vi "addBreak.vi"(8 "error in (no error)":errorcluster, 11 "xwpfRun.PageBreak in":refnum<class "xwpfRun.PageBreak.lvclass">) -> (0 "error out":errorcluster, 3 "xwpfRun.PageBreak out":refnum<class "xwpfRun.PageBreak.lvclass">)   [LabVIEW 2017, in "Word_Specific.lvlib" / "xwpfRun.PageBreak.lvclass"]
uses:
  xwpfRun.PageBreak.lvclass
  C:/Users/Neo/Desktop/Dev_Tools_BR/LabVIEW_NPOI/src/LabVIEW NPOI/xwpfRun/xwpfRun.lvclass
  xwpfRun/xwpfRun.lvclass/xwpfRun.ctl
  C:/Users/Neo/Desktop/Dev_Tools_BR/LabVIEW_NPOI/src/lib/NPOI 2.1.1/NPOI.OOXML.dll
  lib/NPOI 2.1.1/NPOI.OOXML.dll
  xwpfRun/Get Run Ref.vi
  xwpfRun.Normal/xwpfRun.Normal.lvclass
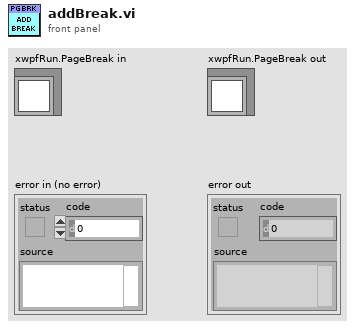
[diagram p1: front panel]
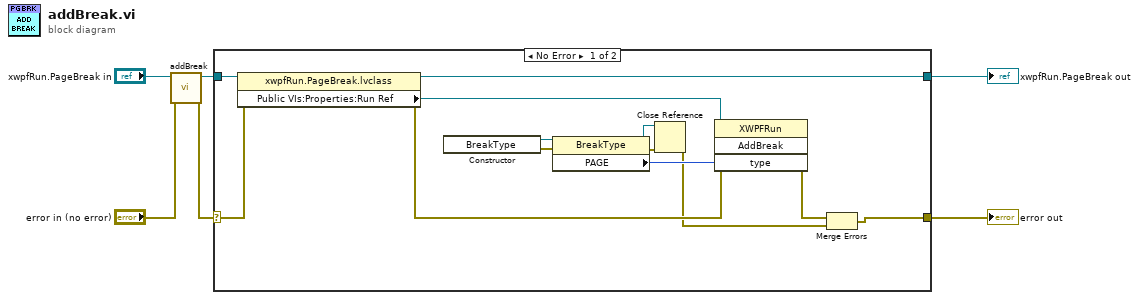
[diagram p0: block diagram]
diagram:
  n1 = call-parent "addBreak.vi"("error in (no error)"="error in (no error)", "xwpfRun in"="xwpfRun.PageBreak in") -> ("error out"=w4:errorcluster, "xwpfRun out"=w2:refnum<class "xwpfRun.PageBreak.lvclass">)  [unwired: 8 in]
  n2 = case shown="No Error" w4 {
    selector: w4 -> [w17 w21]
    tunnel: [w8 w21] -> w3
    tunnel: w2 -> [w19 w20]
    tunnel: [w18 w20] -> w1
    frame No Error {
      n3 = property class="xwpfRun.PageBreak.lvclass"(reference=w19, error in=w17) -> (reference out=w18:refnum<class "xwpfRun.PageBreak.lvclass">, error out=w15:errorcluster, "Public VIs:Properties:Run Ref"=w16:refnum<k24>)
      n4 = constructor class="BreakType"() -> (reference out=w13:refnum<k24>, error out=w12:errorcluster)  [unwired: 3 in, 1 out]
      n5 = property class="BreakType"(reference=w13, error in=w12) -> (reference out=w9:refnum<k24>, error out=w10:errorcluster, "PAGE"=w11:i32)
      n6 = Close Reference(reference=w9, error in (no error)=w10) -> (error out=w7:errorcluster)
      n7 = invoke class="XWPFRun" method="AddBreak"(reference=w16, error in=w15, "type"=w11) -> (error out=w14:errorcluster)  [unwired: 1 in, 3 out]
      n8 = Merge Errors(w14, w7) -> (w8:errorcluster)
    }
    frame Error {
    }
  }
  "error out" <- w3
  "xwpfRun.PageBreak out" <- w1
